vi "Check.vi"(7 "错误输入（无错误）":errorcluster, 8 "长度":i32, 9 "索引":i32, 10 "Array引用":refnum<vi>, 11 "Bool引用":refnum<vi>) -> (3 "错误输出":errorcluster)   [LabVIEW 2011]
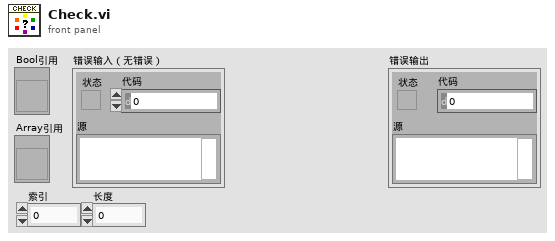
[diagram p1: front panel]
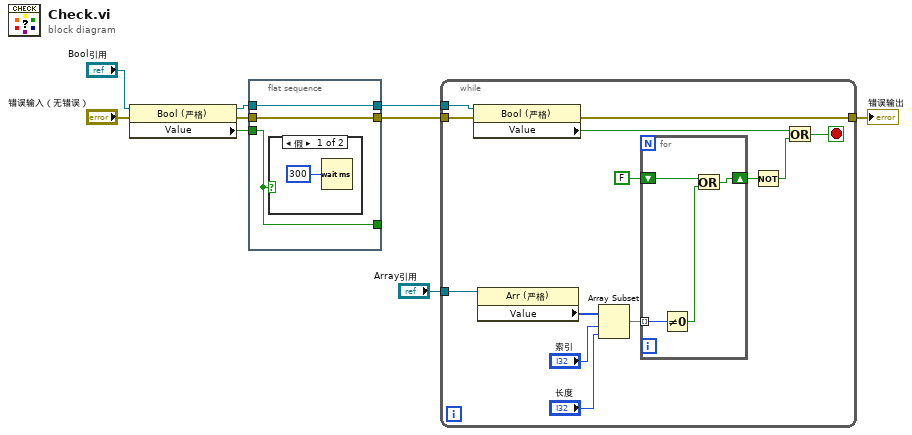
[diagram p0: block diagram]
diagram:
  n1 = property on="属性节点" class="Bool (严格)"(reference="Bool引用", error in="错误输入（无错误）") -> (reference out=w5:refnum<vi>, error out=w6:errorcluster, "Value"=w8:bool)
  n2 = flat-sequence {
    tunnel: w8 -> [w12]
    tunnel: [w12] -> _
    tunnel: w6 -> [w11]
    tunnel: [w11] -> w3
    tunnel: w5 -> [w10]
    tunnel: [w10] -> w4
    frame #0 {
      n3 = case shown="假" w12 {
        frame False {
          n4 = Wait (ms)(milliseconds to wait=u32 300 ("等待时间（毫秒）")) -> ()  [unwired: 1 out]
        }
        frame True {
        }
      }
    }
  }
  n5 = while {
    tunnel: w4 -> [w20]
    tunnel: w3 -> [w19]
    tunnel: "Array引用" -> [w17]
    tunnel: [w16] -> w1
    stop <- w21 stop-if-true
    n6 = property on="属性节点" class="Bool (严格)"(reference=w20, error in=w19) -> (error out=w16:errorcluster, "Value"=w18:bool)  [unwired: 1 out]
    n7 = property on="属性节点" class="Arr (严格)"(reference=w17) -> ("Value"=w25:i32[])  [unwired: 1 in, 2 out]
    n8 = Array Subset(array=w25, index="索引", length="长度") -> (w24:i32[])
    n9 = for {
      shift-right: [w28] -> w23
      shift-left: FALSE -> [w29]
      tunnel: w24 -> [w27] mode=indexing
      n10 = Not Equal To 0?(x=w27) -> (x != 0?=w30:bool)
      n11 = Or(x=w29, y=w30) -> (x .or. y?=w28:bool)
    }
    n12 = Not(x=w23) -> (.not. x?=w22:bool)
    n13 = Or(x=w18, y=w22) -> (x .or. y?=w21:bool)
  }
  "错误输出" <- w1
